vi "database1查询.vi"(6 "时间2":string, 7 "error in (no error)":errorcluster, 8 "table":string, 9 "时间1":string, 10 "database":string="database1.mdb") -> (0 "error out":errorcluster, 1 "database溢出":bool, 2 "data":string[][](table), 3 "recordset data":variant[][](array[variant]))   [LabVIEW 2016, in "数据传输系统-06.lvlib"]
uses:
  <vilib>/Utility/sysdir.llb/System Directory Type.ctl
  <vilib>/addons/database/Connection.llb/DB Tools Open Connec (String).vi
  <vilib>/addons/database/Connection.llb/Conn Execute.vi
  <vilib>/addons/database/Recordset.llb/Rec Fetch Recordset Data (R).vi
  <vilib>/addons/database/Recordset.llb/Rec Destroy - Connection.vi
  <vilib>/addons/database/_DB Variant To Data/Database Variant To Data.xnode
  <vilib>/addons/database/NI_Database_API.lvlib
panel:
  out "SQL query":string
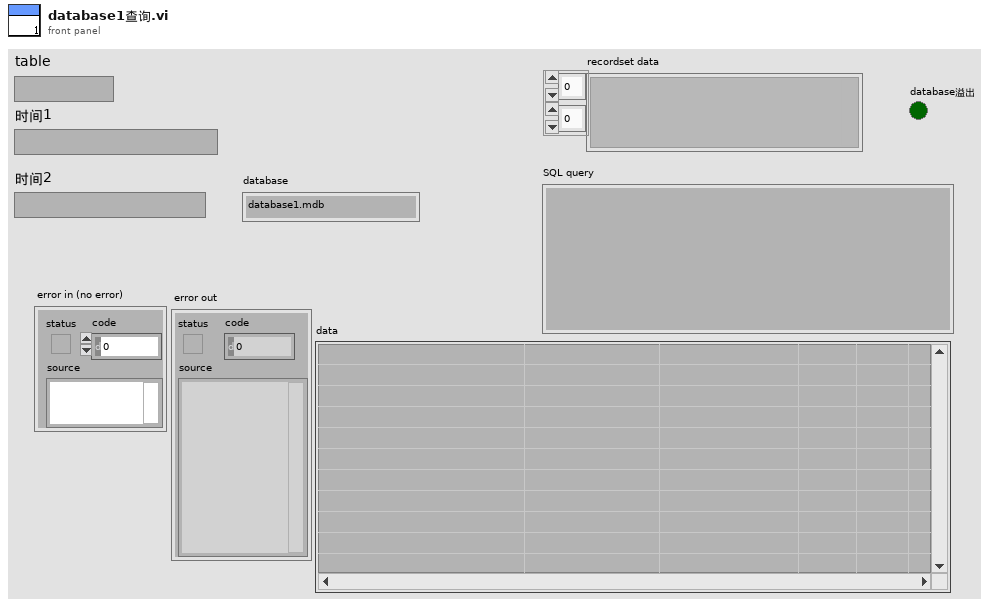
[diagram p1: front panel]
types:
  T1 = typedef "System Directory Type.ctl" = i32
  T2 = typedef "NI_Database_API.lvlib/Conn ObjectReference.ctl" = refnum<k1>
  T3 = typedef "NI_Database_API.lvlib/Rec ObjectReference.ctl" = refnum<k1>
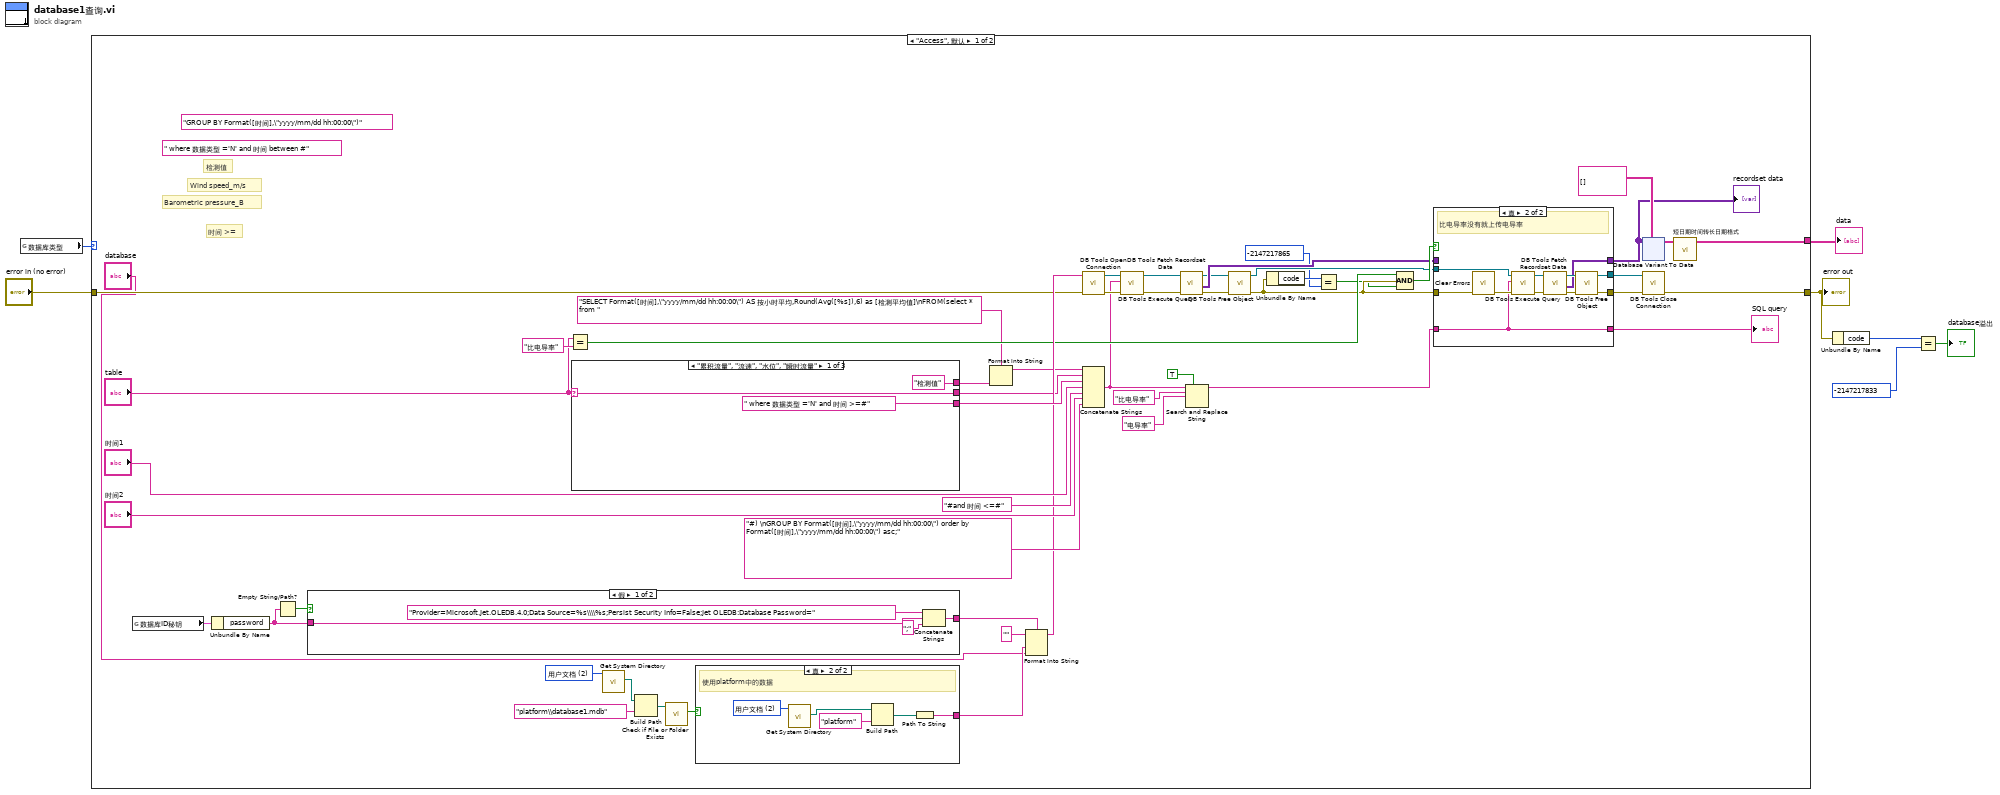
[diagram p0: block diagram]
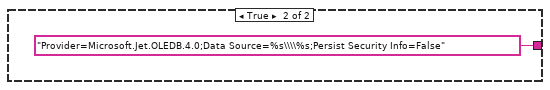
[diagram p2: hidden frame]
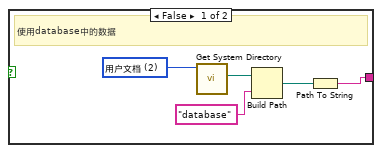
[diagram p4: hidden frame]
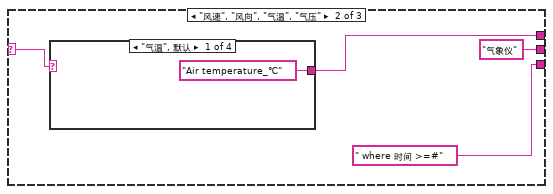
[diagram p5: hidden frame]
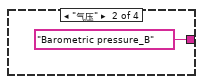
[diagram p6: hidden frame]
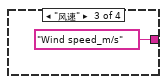
[diagram p7: hidden frame]
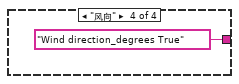
[diagram p8: hidden frame]
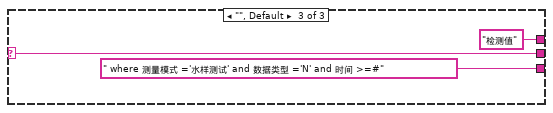
[diagram p9: hidden frame]
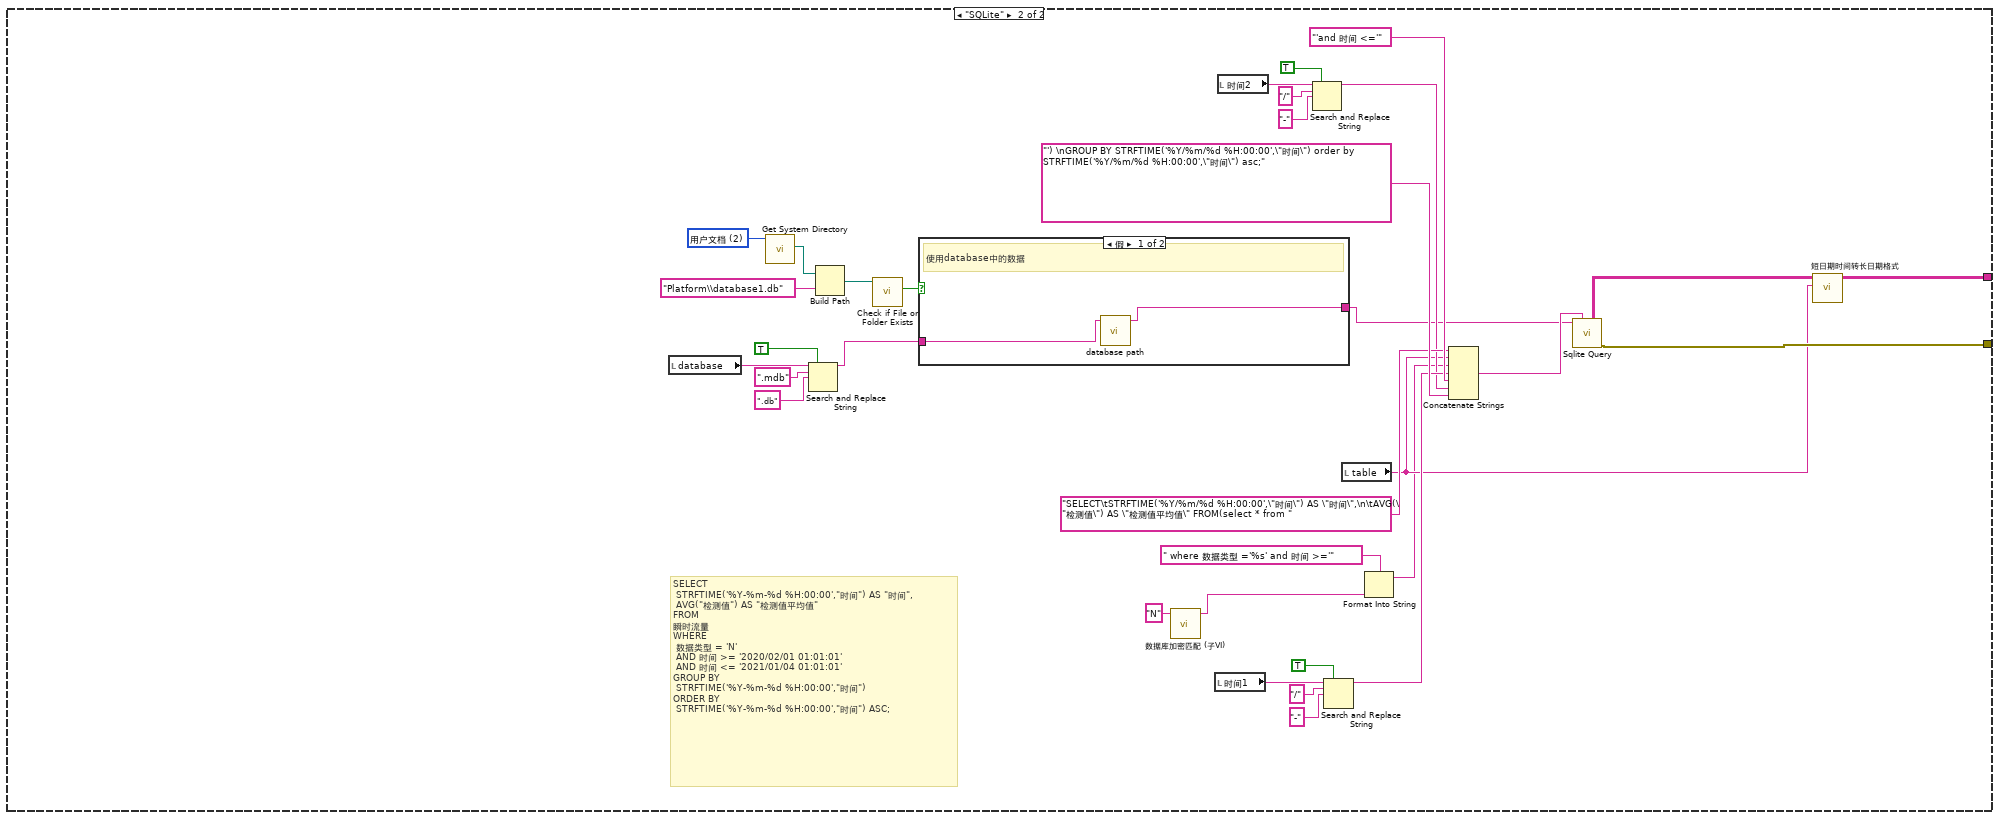
[diagram p10: hidden frame]
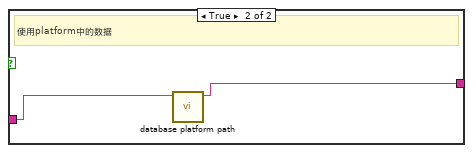
[diagram p11: hidden frame]
diagram:
  n1 = global read "断电保存全局.vi" "数据库类型"() -> (w7:enum16{"Access", "SQLite"})
  n2 = case shown="\"Access\", 默认" w7 {
    tunnel: [w15 w157] -> w4
    tunnel: "error in (no error)" -> [w14 _]
    tunnel: [w9 w173] -> w5
    frame "Access", Default {
      (unwired) " where 数据类型 ='N' and 时间 between #"
      w50 = T1 2 items=["用户目录"=0, "用户桌面"=1, "用户文档"=2, "用户应用程序数据"=3, "用户设置"=4, "用户临时目录"=5, "公共文档"=6, "公共应用程序数据"=7, "公共设置"=8, "公共缓存"=13, "系统核心库"=9, "系统安装库"=10, "应用程序文件"=11, "启动盘根目录"=12] ("system directory type")
      (unwired) "GROUP BY Format([时间],\"yyyy/mm/dd hh:00:00\")"
      # "时间 >="
      # "Wind speed_m/s"
      # "检测值"
      # "Barometric pressure_B"
      n3 = global read "外部交互全局.vi" "数据库ID秘钥"() -> (w16:cluster{"userID":string, "password":string})
      n4 = Unbundle By Name(w16) -> ("password"=w18:string)
      n5 = Empty String/Path?(string/path=w18) -> (empty?=w19:bool)
      n6 = case shown="假" w19 {
        tunnel: [w104 "Provider=Microsoft.Jet.OLEDB.4.0;Data Source=%s\\\\%s;Persist Security Info=False" ("格式字符串")] -> w17
        tunnel: w18 -> [w107 _]
        frame False {
          n7 = Concatenate Strings("Provider=Microsoft.Jet.OLEDB.4.0;Data Source=%s\\\\%s;Persist Security Info=False;Jet OLEDB:Database Password=" ("格式字符串"), w107, ";" ("字符串")) -> (w104:string)
        }
        frame True {
        }
      }
      n8 = Equal?(x="table", y="比电导率") -> (x = y?=w39:bool)
      n9 = case shown="\"累积流量\", \"流速\", \"水位\", \"瞬时流量\"" "table" {
        selector: "table" -> [w135 w138 w146]
        tunnel: [" where 数据类型 ='N' and 时间 >=#" " where 时间 >=#" " where 测量模式 ='水样测试' and 数据类型 ='N' and 时间 >=#"] -> w53
        tunnel: ["检测值" w137 "检测值"] -> w23
        tunnel: [w135 "气象仪" w146] -> w21
        frame "累积流量", "流速", "水位", "瞬时流量" {
        }
        frame "风速", "风向", "气温", "气压" {
          n10 = case shown="\"气温\", 默认" w138 {
            tunnel: ["Air temperature_℃" "Barometric pressure_B" "Wind speed_m/s" "Wind direction_degrees True"] -> w137
            frame "气温", Default {
            }
            frame "气压" {
            }
            frame "风速" {
            }
            frame "风向" {
            }
          }
        }
        frame "", Default {
        }
      }
      n11 = call <vilib>:"Get System Directory.vi"("system directory type"=w50) -> ("system directory"=w51:path)  [unwired: 10 in]
      n12 = Build Path(base path=w51, name or relative path="platform\\database1.mdb" ("condition")) -> (appended path=w49:path)
      n13 = call <vilib>:"Check if File or Folder Exists.vi"("path"=w49) -> ("file or folder exists?"=w47:bool)  [unwired: 8 in, 2 out]
      n14 = case shown="真" w47 {
        tunnel: [w124 w129] -> w46
        frame False {
          w127 = T1 2 items=["用户目录"=0, "用户桌面"=1, "用户文档"=2, "用户应用程序数据"=3, "用户设置"=4, "用户临时目录"=5, "公共文档"=6, "公共应用程序数据"=7, "公共设置"=8, "公共缓存"=13, "系统核心库"=9, "系统安装库"=10, "应用程序文件"=11, "启动盘根目录"=12] ("system directory type")
          # "使用database中的数据"
          n15 = call <vilib>:"Get System Directory.vi"("system directory type"=w127) -> ("system directory"=w126:path)  [unwired: 10 in]
          n16 = Build Path(base path=w126, name or relative path="database" ("condition")) -> (appended path=w128:path)
          n17 = Path To String(path=w128) -> (string=w124:string)
        }
        frame True {
          w133 = T1 2 items=["用户目录"=0, "用户桌面"=1, "用户文档"=2, "用户应用程序数据"=3, "用户设置"=4, "用户临时目录"=5, "公共文档"=6, "公共应用程序数据"=7, "公共设置"=8, "公共缓存"=13, "系统核心库"=9, "系统安装库"=10, "应用程序文件"=11, "启动盘根目录"=12] ("system directory type")
          # "使用platform中的数据"
          n18 = call <vilib>:"Get System Directory.vi"("system directory type"=w133) -> ("system directory"=w132:path)  [unwired: 10 in]
          n19 = Build Path(base path=w132, name or relative path="platform" ("condition")) -> (appended path=w130:path)
          n20 = Path To String(path=w130) -> (string=w129:string)
        }
      }
      n21 = Format Into String(format string="SELECT Format([时间],\"yyyy/mm/dd hh:00:00\") AS 按小时平均,Round(Avg([%s]),6) as [检测平均值]\nFROM(select * from ", w23) -> (resulting string=w20:string)  [unwired: 2 in, 1 out]
      n22 = Format Into String(format string=w17, initial string="" ("初始字符串"), w46, "database") -> (resulting string=w45:string)  [unwired: 1 in, 1 out]
      n23 = call-poly <vilib>:"DB Tools Open Connection.vi"("error in (no error)"=w14, "connection information"=w45) -> ("error out"=w58:errorcluster, "connection reference"=w41:T2)  [unwired: 6 in]
      n24 = Concatenate Strings(w20, w21, w53, "时间1", "#and 时间 <=#", "时间2", "#) \nGROUP BY Format([时间],\"yyyy/mm/dd hh:00:00\") order by Format([时间],\"yyyy/mm/dd hh:00:00\") asc;" ("字符串")) -> (w30:string)
      n25 = call-poly <vilib>:"DB Tools Execute Query.vi"("error in (no error)"=w58, "SQL query"=w30, "connection reference"=w41) -> ("error out"=w37:errorcluster, "recordset reference"=w42:T3)  [unwired: 5 in]
      n26 = call-poly <vilib>:"DB Tools Fetch Recordset Data.vi"("error in (no error)"=w37, "recordset reference"=w42) -> ("error out"=w59:errorcluster, "recordset data"=w43:variant[][], "recordset reference out"=w38:T3)  [unwired: 3 in]
      n27 = Search and Replace String(replace all?=TRUE ("替换全部？(F)"), input string=w30, search string="比电导率" ("搜索字符串"), replace string="电导率" ("替换字符串(\"\")")) -> (result string=w27:string)  [unwired: 4 in, 3 out]
      n28 = call-poly <vilib>:"DB Tools Free Object.vi"("error in (no error)"=w59, "recordset reference"=w38) -> ("error out"=w32:errorcluster, "connection reference"=w36:T2)  [unwired: 8 in]
      n29 = Unbundle By Name(w32) -> ("code"=w34:i32)
      n30 = Equal?(x=w34, y=-2147217865 ("code")) -> (x = y?=w31:bool)
      n31 = Compound Arithmetic op=AND ("复合运算")(w39, w32, w31) -> (w44:bool)
      n32 = case shown="真" w44 {
        tunnel: w27 -> [w109 w113]
        tunnel: w36 -> [w110 w118]
        tunnel: [w110 w114] -> w35
        tunnel: [w112 w116] -> w10
        tunnel: w43 -> [w112 _]
        tunnel: w32 -> [w111 w123]
        tunnel: [w111 w115] -> w11
        tunnel: [w109 w113] -> w25
        frame False {
        }
        frame True {
          # "比电导率没有就上传电导率"
          n33 = call <vilib>:"Clear Errors.vi"("error in (no error)"=w123) -> ("error out"=w117:errorcluster)  [unwired: 5 in, 1 out]
          n34 = call-poly <vilib>:"DB Tools Execute Query.vi"("error in (no error)"=w117, "SQL query"=w113, "connection reference"=w118) -> ("error out"=w119:errorcluster, "recordset reference"=w121:T3)  [unwired: 5 in]
          n35 = call-poly <vilib>:"DB Tools Fetch Recordset Data.vi"("error in (no error)"=w119, "recordset reference"=w121) -> ("error out"=w122:errorcluster, "recordset data"=w116:variant[][], "recordset reference out"=w120:T3)  [unwired: 3 in]
          n36 = call-poly <vilib>:"DB Tools Free Object.vi"("error in (no error)"=w122, "recordset reference"=w120) -> ("error out"=w115:errorcluster, "connection reference"=w114:T2)  [unwired: 8 in]
        }
      }
      "SQL query" <- w25
      "recordset data" <- w10
      n37 = xnode "Database Variant To Data"("database variant"=w10, "type"=string[][] []) -> ("data"=w12:string[][])  [unwired: 1 in, 1 out]
      n38 = call <vilib>:"DB Tools Close Connection.vi"("error in (no error)"=w11, "connection reference"=w35) -> ("error out"=w15:errorcluster)  [unwired: 5 in]
      n39 = call "短日期时间转长日期格式.vi"("data"=w12) -> ("输出数组"=w9:string[][])  [unwired: 10 in]
    }
    frame "SQLite" {
      w177 = T1 2 items=["用户目录"=0, "用户桌面"=1, "用户文档"=2, "用户应用程序数据"=3, "用户设置"=4, "用户临时目录"=5, "公共文档"=6, "公共应用程序数据"=7, "公共设置"=8, "公共缓存"=13, "系统核心库"=9, "系统安装库"=10, "应用程序文件"=11, "启动盘根目录"=12] ("system directory type")
      # "SELECT\n\tSTRFTIME('%Y-%m-%d %H:00:00',\"时间\") AS \"时间\",\n\tAVG(\"检测值\") AS \"检测值平均值\"\nFROM\n瞬时流量 \nWHERE\n\t数据类型 = 'N' \n\tAND 时间 >= '2020/02/01 01:01:01' \n\tAND 时间 <= '2021/01/04 01:01:01' \nGROUP BY\n\tSTRFTIME('%Y-%m-%d %H:00:00',\"时间\")\nORDER BY\n\tSTRFTIME('%Y-%m-%d %H:00:00',\"时间\") ASC;"
      n40 = local read "database"() -> (w158:string)
      n41 = call <vilib>:"Get System Directory.vi"("system directory type"=w177) -> ("system directory"=w176:path)  [unwired: 10 in]
      n42 = Search and Replace String(replace all?=TRUE ("替换全部？(F)"), input string=w158, search string=".mdb" ("搜索字符串"), replace string=".db" ("替换字符串(\"\")")) -> (result string=w149:string)  [unwired: 4 in, 3 out]
      n43 = Build Path(base path=w176, name or relative path="Platform\\database1.db" ("condition")) -> (appended path=w178:path)
      n44 = call <vilib>:"Check if File or Folder Exists.vi"("path"=w178) -> ("file or folder exists?"=w180:bool)  [unwired: 8 in, 2 out]
      n45 = case shown="假" w180 {
        tunnel: [w181 w183] -> w148
        tunnel: w149 -> [w182 w184]
        frame False {
          # "使用database中的数据"
          n46 = call "database path.vi"("database"=w182) -> ("Path out"=w181:string)  [unwired: 9 in, 1 out]
        }
        frame True {
          # "使用platform中的数据"
          n47 = call "database platform path.vi"("database"=w184) -> ("Path out"=w183:string)  [unwired: 10 in]
        }
      }
      n48 = call "数据库加密匹配 (子VI).vi"("输入参数"="N") -> ("Encoded String"=w151:string)  [unwired: 10 in]
      n49 = local read "时间1"() -> (w165:string)
      n50 = local read "时间2"() -> (w163:string)
      n51 = Search and Replace String(replace all?=TRUE ("替换全部？(F)"), input string=w163, search string="/" ("搜索字符串"), replace string="-" ("替换字符串(\"\")")) -> (result string=w162:string)  [unwired: 4 in, 3 out]
      n52 = Search and Replace String(replace all?=TRUE ("替换全部？(F)"), input string=w165, search string="/" ("搜索字符串"), replace string="-" ("替换字符串(\"\")")) -> (result string=w164:string)  [unwired: 4 in, 3 out]
      n53 = local read "table"() -> (w155:string)
      n54 = Format Into String(format string=" where 数据类型 ='%s' and 时间 >='", w151) -> (resulting string=w153:string)  [unwired: 2 in, 1 out]
      n55 = Concatenate Strings("SELECT\tSTRFTIME('%Y/%m/%d %H:00:00',\"时间\") AS \"时间\",\n\tAVG(\"检测值\") AS \"检测值平均值\" FROM(select * from ", w155, w153, w164, "'and 时间 <='", w162, "') \nGROUP BY STRFTIME('%Y/%m/%d %H:00:00',\"时间\") order by STRFTIME('%Y/%m/%d %H:00:00',\"时间\") asc;" ("字符串")) -> (w150:string)
      n56 = call "Sqlite Query.vi"("DB Path"=w148, "SQL Query"=w150) -> ("Results"=w156:string[][], "error out"=w157:errorcluster)  [unwired: 11 in, 1 out]
      n57 = call "短日期时间转长日期格式.vi"("table输入"=w155, "data"=w156) -> ("输出数组"=w173:string[][])  [unwired: 9 in]
    }
  }
  "error out" <- w4
  "data" <- w5
  n58 = Unbundle By Name(w4) -> ("code"=w3:i32)
  n59 = Equal?(x=w3, y=-2147217833 ("code")) -> (x = y?=→"database溢出":bool)
